vi "Draw ROI on Line Scan Display.vi"(7 "Draw ROI on Line Scan Display_Command":T1, 8 "error in (no error)":errorcluster) -> (0 "error out":errorcluster)   [LabVIEW 2012]
doc: "SciScan 1.2 160622"
uses:
  Draw ROI on Line Scan Display Command.ctl
  GFG/GFGDisplayRefsGet.vi
  GFG/GFG library.lvlib
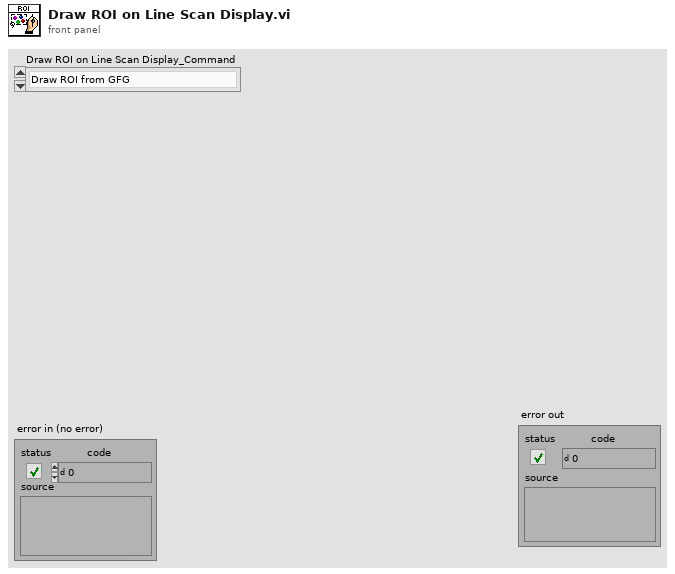
[diagram p1: front panel]
types:
  T1 = typedef "Draw ROI on Line Scan Display Command.ctl" = enum16{"Draw ROI from GFG", "Clear ROI"}
  T2 = cluster{"Global Rectangle":i32[], "Contours":cluster{"Contour Type":u32, "ROI Type":u32, "Points":i32[]}[]}
  T3 = typedef "ROI Descriptor" = cluster{"Global Rectangle":i32[], "Contours":cluster{"ID":enum32{"External", "Internal"}, "Type":u32, "Coordinates":i32[]}[]}
  T4 = cluster{"Channel 1 small":refnum<vi>, "Channel 2 small":refnum<vi>, "Channel 3 small":refnum<vi>, "Channel 4 small":refnum<vi>, "Channel 1 large":refnum<vi>, "Channel 2 large":refnum<vi>, "Channel 3 large":refnum<vi>, "Channel 4 large":refnum<vi>, "RGB overlay":refnum<vi>, "ROI Image display":refnum<vi>, "arb line scan display":refnum<vi>, "Channel 5 large":refnum<vi>}
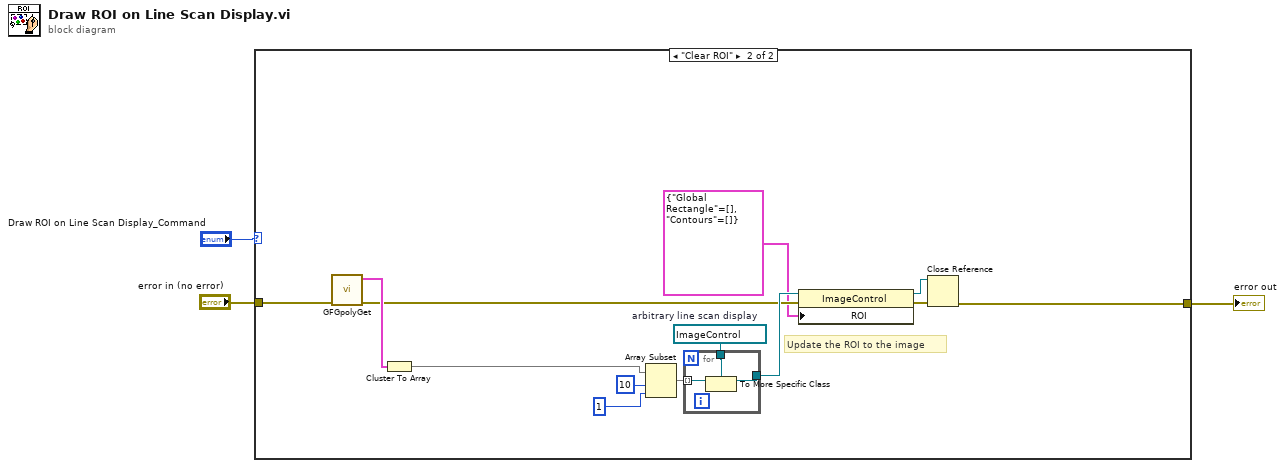
[diagram p0: block diagram]
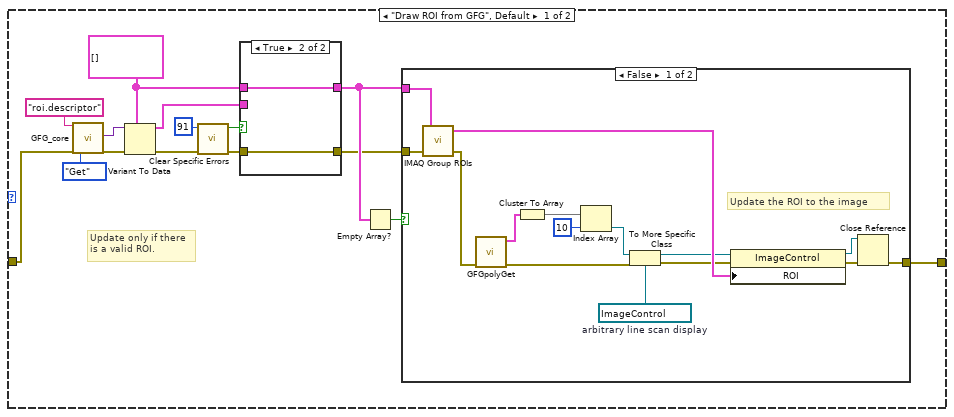
[diagram p2: hidden frame]
diagram:
  n1 = case shown="\"Clear ROI\"" "Draw ROI on Line Scan Display_Command" {
    tunnel: "error in (no error)" -> [w14 w40]
    tunnel: [w15 w39] -> w2
    frame "Draw ROI from GFG", Default {
      w8 = T3[] []
      # "Update only if there is a valid ROI."
      n2 = call "GFG_core.vi"("Variable Name in"="roi.descriptor", "error in (no error)"=w14, "Action"=enum16{"Init", "Set", "Get"}."Get") -> ("Variant Out"=w16:variant, "error out"=w13:errorcluster)  [unwired: 10 in, 5 out]
      n3 = Variant To Data(error in=w13, type=w8, Variant=w16) -> (data=w6:T3[], error out=w11:errorcluster)
      n4 = call "Clear Specific Errors.vi"("Error In"=w11, "Error number In"=91) -> ("Error Out"=w5:errorcluster, "Error Cleared?"=w9:bool)  [unwired: 8 in]
      n5 = case shown="True" w9 {
        tunnel: w8 -> [_ w22]
        tunnel: [w20 w22] -> w7
        tunnel: w6 -> [w20 _]
        tunnel: w5 -> [w19 w21]
        tunnel: [w19 w21] -> w4
        frame False {
        }
        frame True {
        }
      }
      n6 = Empty Array?(array=w7) -> (empty?=w12:bool)
      n7 = case shown="False" w12 {
        tunnel: w4 -> [w37 w38]
        tunnel: w7 -> [w31 _]
        tunnel: [w30 w38] -> w15
        frame False {
          w32 = refnum<vi> refnum  # arbitrary line scan display
          # "Update the ROI to the image"
          n8 = call "IMAQ Group ROIs"("error in (no error)"=w37, "ROI Descriptors"=w31) -> ("error out"=w25:errorcluster, "ROI Descriptor out"=w34:T3)  [unwired: 2 in]
          n9 = call-poly "GFGpolyGet.vi"("error in (no error)"=w25) -> ("error out"=w24:errorcluster, "DisplayRefsOut(generic class)"=w33:T4)  [unwired: 9 in]
          n10 = Cluster To Array(cluster=w33) -> (array=w29:refnum<vi>[])
          n11 = Index Array(array=w29, index=10) -> (element=w27:refnum<vi>)
          n12 = To More Specific Class(target class=w32, reference=w27, error in=w24) -> (specific class reference=w26:refnum<vi>, error out=w23:errorcluster)
          n13 = property class="ImageControl"(reference=w26, error in=w23, "ROI"=w34) -> (reference out=w35:refnum<vi>, error out=w36:errorcluster)
          n14 = Close Reference(reference=w35, error in (no error)=w36) -> (error out=w30:errorcluster)
        }
        frame True {
        }
      }
    }
    frame "Clear ROI" {
      w46 = refnum<vi> refnum  # arbitrary line scan display
      # "Update the ROI to the image"
      n15 = call-poly "GFGpolyGet.vi"("error in (no error)"=w40) -> ("error out"=w44:errorcluster, "DisplayRefsOut(generic class)"=w45:T4)  [unwired: 9 in]
      n16 = Cluster To Array(cluster=w45) -> (array=w48:refnum<vi>[])
      n17 = Array Subset(array=w48, index=10, length=1) -> (w47:refnum<vi>[])
      n18 = for {
        tunnel: w47 -> [w54] mode=indexing
        tunnel: w46 -> [w53]
        tunnel: [w52] -> w51
        n19 = To More Specific Class(target class=w53, reference=w54) -> (specific class reference=w52:refnum<vi>)  [unwired: 1 in, 1 out]
      }
      n20 = property class="ImageControl"(reference=w51, error in=w44, "ROI"=T2 {"Global Rectangle"=[], "Contours"=[]}) -> (reference out=w41:refnum<vi>, error out=w42:errorcluster)
      n21 = Close Reference(reference=w41, error in (no error)=w42) -> (error out=w39:errorcluster)
    }
  }
  "error out" <- w2
